vi "Check Status.vi"(8 "error in (no error)":errorcluster, 11 "Instrument in":refnum<class "Instrument.lvclass">) -> (0 "error out":errorcluster, 1 "Status":string, 2 "Ready?":bool, 3 "Instrument out":refnum<class "Instrument.lvclass">)   [LabVIEW 2017, in "Instrument.lvclass"]
doc: "(Dynamic) Check if the instrument is powered on and update its member fields with the instrument's current status. Optionally return a text status message."
uses:
  Instrument.lvclass
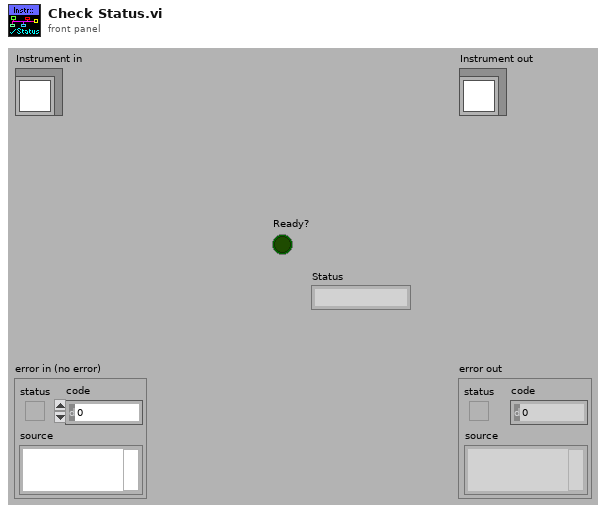
[diagram p1: front panel]
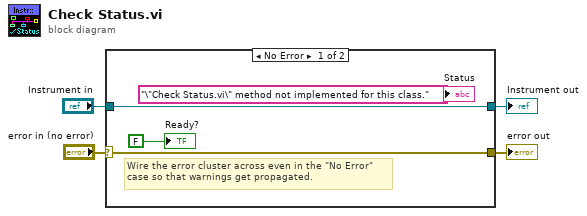
[diagram p0: block diagram]
diagram:
  n1 = case shown="No Error" "error in (no error)" {
    selector: "error in (no error)" -> [w7 w10]
    tunnel: [w7 w10] -> w3
    tunnel: [w8 w9] -> w1
    tunnel: "Instrument in" -> [w8 w9]
    frame No Error {
      # "Wire the error cluster across even in the \"No Error\"\ncase so that warnings get propagated."
      "Ready?" <- FALSE ("Ready?")
      "Status" <- "\"Check Status.vi\" method not implemented for this class." ("Status")
    }
    frame Error {
    }
  }
  "error out" <- w3
  "Instrument out" <- w1
